vi "Test motor controll ability.vi"() -> ()   [LabVIEW 2016]
uses:
  Default PDO conf.ctl
  <vilib>/userdefined/High Color/nirio_resource_hc.ctl
  <vilib>/Platform/TimedLoop/XDataNode/timing_clust.ctl
  <vilib>/Platform/TimedLoop/XDataNode/nitl_modes.ctl
  <vilib>/Platform/TimedLoop/XDataNode/wakeup.ctl
  <vilib>/FPGAPlugInAG/cRIO-9033/niLvFpga_Open_cRIO-9033.vi
  <vilib>/rvi/interface/common/dynamic/niFpgaDynamicAddResources.vi
  <vilib>/CANopenLib/CANOPEN.llb/CANopen Emergency Create.vi
  <vilib>/CANopenLib/CANOPEN.llb/CANopen SDO Create.vi
  Set mode of operation.vi
  Set control mode.vi
  <vilib>/CANopenLib/CANOPEN.llb/CANopen SDO Close.vi
  Set Speed or Torque.vi
  Get Error.vi
  <vilib>/CANopenLib/CANOPEN.llb/CANopen Interface Close.vi
  <vilib>/rvi/interface/nirviOpenFPGA/nirviOpenFPGA.xnode
  FPGA Bitfiles/project_FPGATarget_FPGAMain_kDJZXzfRsH0.lvbitx
  Program Files (x86)/National Instruments/LabVIEW 2016/examples/robotics/EPOS2 CANOpen Driver/FPGA/FPGA Main.vi
  <vilib>/Platform/TimedLoop/XDataNode/XDataNode.xnode
  <vilib>/Platform/TimedLoop/XDataNode/XDNodeRunTimeDep.lvlib
panel:
  out "x+1":u16
  out "Used Node ID":u8 min=1 max=127 step=1
  in  "Node ID Left":u8=1 min=1 max=127 step=1
  in  "?":enum32{"Setup", "Operation", "Debug"}(tab)
  in  "Mode of operation":i8(ring)=9 items=["Induction VF – testing purposes only"=-5, "Aligning rotor position"=-4, "Current stepper – testing purposes only "=-3, "Voltage stepper – testing purposes only"=-2, "Voltage constant angle – testing purposes only"=-1, "No mode"=0, "Cyclic sync position"=8, "Cyclic sync velocity"=9, "Cyclic sync torque"=10]
  in  "Control Mode":u8(ring)=2 items=["Velocity"=2, "Torque"=1]
  out "Waveform Chart":cluster{"Controller temp":u8, "Motor temp":u8}(graph)
  in  "Set":bool
  in  "Stop":bool
  out "Decoded PDO":T1 {"Status word" format="%b"}
  in  "Speed-Torque":i32(knob) scale=-200.0..200.0
  in  "error in (no error)":errorcluster
  out "PDO 1":u8[](array[numeric])
  out "PDO 2":u8[](array[numeric])
  out "PDO 3":u8[](array[numeric])
  out "PDO 4":u8[](array[numeric])
  out "error out":errorcluster
  out "Error code":u16 format="%x"
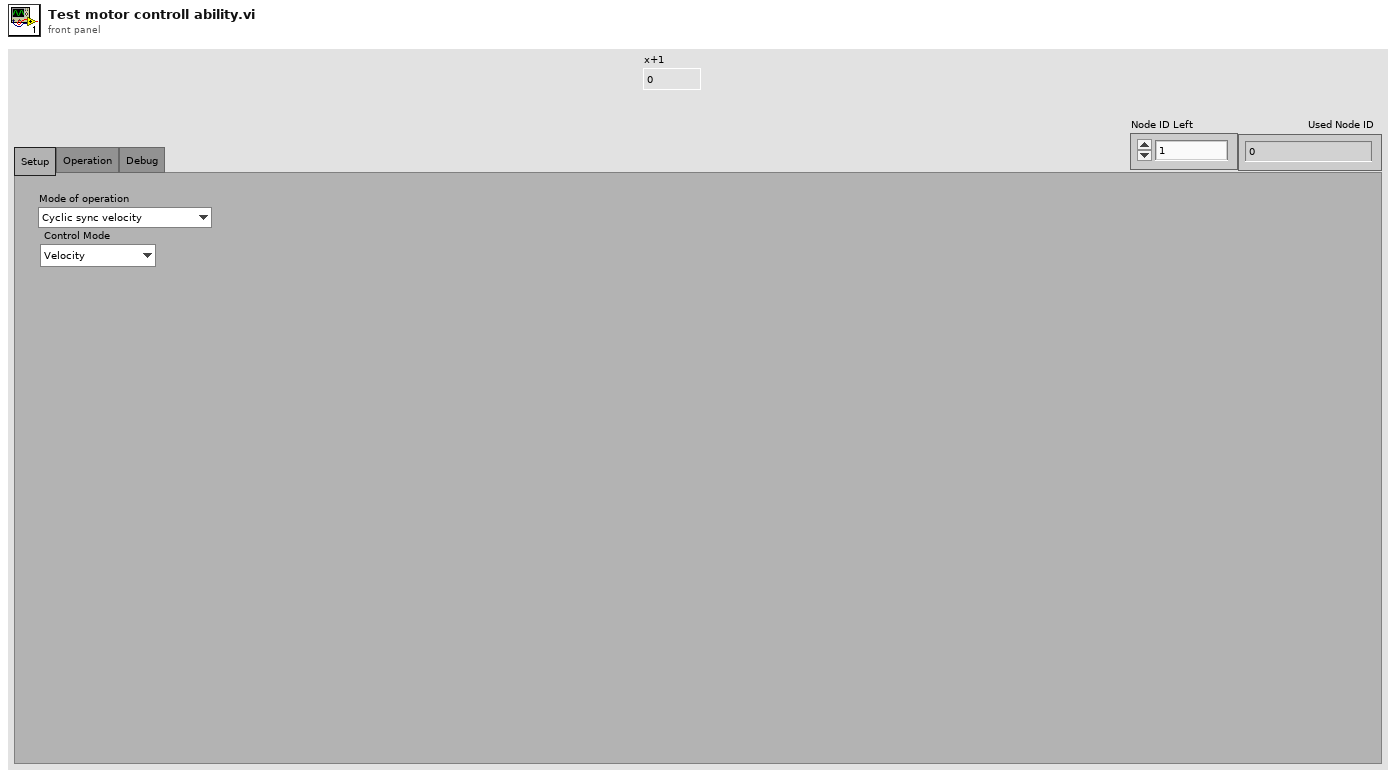
[diagram p1: front panel]
types:
  T1 = typedef "Default PDO conf.ctl" = cluster{"Status word":u16, "Position Actual Value":u32, "Torque Actual Value":u16, "Logic Power Supply Voltage":u16, "Current Demand":i32, "Controller temp":u8, "Motor temp":u8, "DC Link Voltage":u16, "Motor current actual value":u16, "Electrical angle":u16, "Phase A Current":u16, "Phase B Current":u16}
  T2 = typedef "nirio_resource_hc.ctl" = tag
  T3 = typedef "XDNodeRunTimeDep.lvlib/timing_clust.ctl" = cluster{"Expected End [f-1]":u64, "Actual End [f-1]":u64, "Finished Late? [f-1]":bool, "Expected End [i-1]":u64, "Actual End [i-1]":u64, "Finished Late? [i-1]":bool, "Expected Start [i]":u64, "Actual Start [i]":u64, "Expected Start [f]":u64, "Actual Start [f]":u64, "Source Name":string, "Structure Name":string, "Period":i64, "Deadline":i64, "Offset":i64, "Start":i64, "Priority":i32, "Timeout":i32, "Mode":T4, "Wakeup Reason":T5, "Error":errorcluster, "Source Type":string, "Secondary Source Type":string, "Global End Time":u64, "Global Start Time":u64, "Frame Duration":u64, "Iteration Duration":u64, "Assigned CPU":i32, "I/O Scan Engine Mode":u32}
  T4 = typedef "XDNodeRunTimeDep.lvlib/nitl_modes.ctl" = enum32{"No Change", "Process missed periods, maintain original phase", "Discard missed periods, maintain original phase", "Process missed periods, ignore original phase", "Discard missed periods, ignore original phase"}
  T5 = typedef "XDNodeRunTimeDep.lvlib/wakeup.ctl" = enum32{"Normal", "Aborted", "Asynchronous wakeup", "Timing source error", "Timed loop error", "Timeout"}
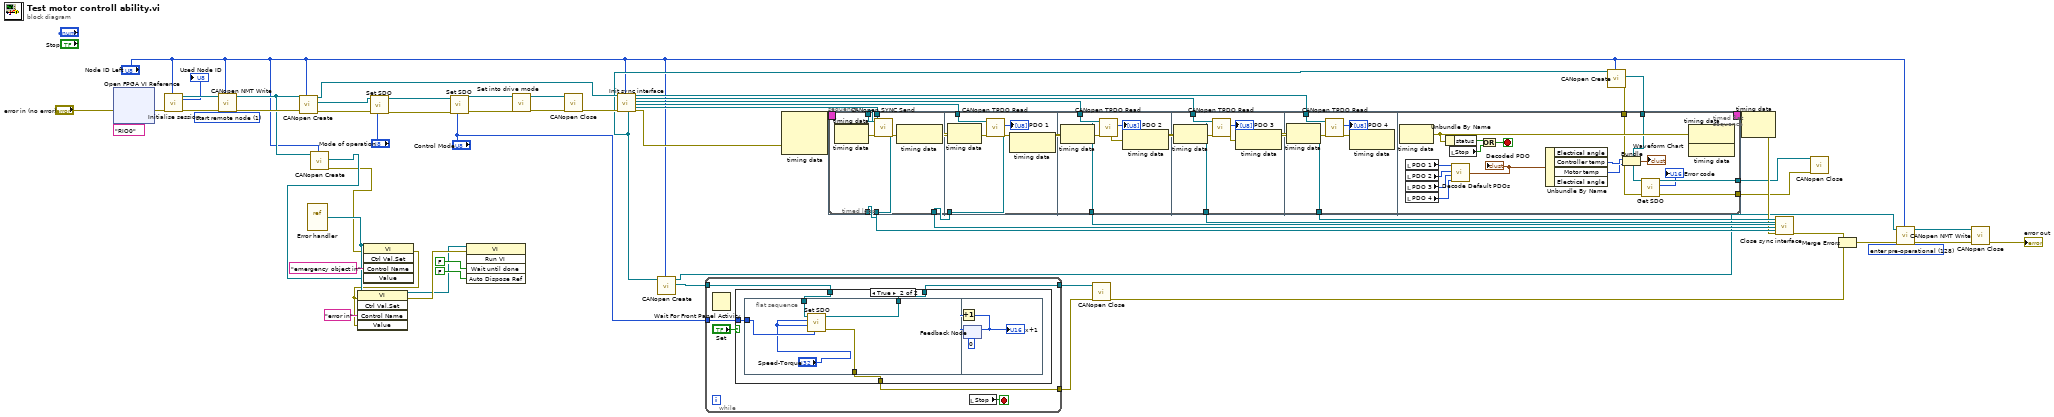
[diagram p0: block diagram]
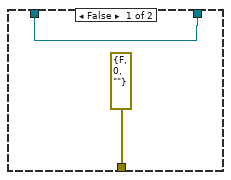
[diagram p2: hidden frame]
diagram:
  w51 = u16 1 items=["start remote node"=1, "stop remote node"=2, "enter pre-operational"=128, "reset node"=129, "reset communication"=130] ("command")
  w57 = u16 128 items=["start remote node"=1, "stop remote node"=2, "enter pre-operational"=128, "reset node"=129, "reset communication"=130] ("command")
  n1 = xnode ("Open FPGA VI Reference")("error in"="error in (no error)", "resource name"=T2 "RIO0") -> ("error out"=w61:errorcluster)  [unwired: 1 out]
  n2 = call "Initialise session.vi"("Node ID"="Node ID Left", "error in"=w61) -> ("error out"=w53:errorcluster, "interface object out"=w52:refnum<k20>, "Used Node ID"=→"Used Node ID":u8)  [unwired: 7 in]
  n3 = call <vilib>:"CANopen NMT Write.vi"("node-ID (0)"="Node ID Left", "error in (no error)"=w53, "command"=w51, "interface object in"=w52) -> ("error out"=w50:errorcluster, "interface object out"=w33:refnum<k20>)  [unwired: 6 in]
  n4 = call-poly <vilib>:"CANopen Create.vi"("node-ID"="Node ID Left", "error in (no error)"=w50, "interface object in"=w33) -> ("error out"=w29:errorcluster, "SDO object out"=w28:refnum<k20>, "interface object out"=w40:refnum<k20>)  [unwired: 6 in]
  n5 = vi-ref "Error handler.vi"() -> (w18:refnum<vi>)
  n6 = call-poly <vilib>:"CANopen Create.vi"("node-ID"="Node ID Left", "interface object in"=w33) -> ("error out"=w13:errorcluster, "emergency object out"=w14:refnum<k20>)  [unwired: 7 in, 1 out]
  n7 = invoke class="VI" method="Ctrl Val.Set"(reference=w18, error in=w13, "Control Name"="emergency object in", "Value"=w14) -> (error out=w17:errorcluster)  [unwired: 1 in, 4 out]
  n8 = invoke class="VI" method="Ctrl Val.Set"(reference=w18, error in=w17, "Control Name"="error in", "Value"=w17) -> (reference out=w15:refnum<vi>, error out=w16:errorcluster)  [unwired: 1 in, 3 out]
  n9 = call-poly "Set SDO.vi"("Mode of operation"="Mode of operation", "error in (no error)"=w29, "SDO object in"=w28) -> ("error out"=w26:errorcluster, "SDO object out"=w27:refnum<k20>)  [unwired: 6 in, 1 out]
  n10 = call-poly "Set SDO.vi"("Control Mode"="Control Mode", "error in (no error)"=w26, "SDO object in"=w27) -> ("error out"=w25:errorcluster, "SDO object out"=w24:refnum<k20>)  [unwired: 6 in, 1 out]
  n11 = invoke class="VI" method="Run VI"(reference=w15, error in=w16, "Wait until done"=FALSE ("Wait Until Done"), "Auto Dispose Ref"=FALSE ("Auto Dispose Reference")) -> ()  [unwired: 1 in, 5 out]
  n12 = call "Set into drive mode.vi"("error in (no error)"=w25, "SDO object in"=w24) -> ("error out"=w49:errorcluster, "SDO object out"=w48:refnum<k20>)  [unwired: 8 in]
  n13 = call-poly <vilib>:"CANopen Close.vi"("error in (no error)"=w49, "SDO object in"=w48) -> ("error out"=w41:errorcluster)  [unwired: 9 in]
  n14 = call "Init sync interface.vi"("interface object in"=w40, "error in (no error)"=w41, "node-ID"="Node ID Left") -> ("interface object out"=w8:refnum<k20>, "TPDO 4 object out"=w7:refnum<k20>, "TPDO 3 object out"=w43:refnum<k20>, "TPDO 2 object out"=w44:refnum<k20>, "TPDO 1 object out"=w45:refnum<k20>, "SYNC object out"=w46:refnum<k20>, "error out"=w42:errorcluster)  [unwired: 10 in]
  n15 = call-poly <vilib>:"CANopen Create.vi"("node-ID"="Node ID Left", "interface object in"=w8) -> ("SDO object out"=w3:refnum<k20>, "interface object out"=w30:refnum<k20>)  [unwired: 7 in, 1 out]
  n16 = while {
    tunnel: [w66] -> w5
    tunnel: w3 -> [w65]
    tunnel: [w64] -> w4
    tunnel: "Control Mode" -> [w63]
    stop <- w68 stop-if-true
    n17 = Wait For Front Panel Activity() -> ()  [unwired: 3 in, 1 out]
    n18 = case shown="True" "Set" {
      tunnel: [errorcluster {"status"=FALSE, "code"=0, "source"=""} ("error out") w74] -> w66
      tunnel: w65 -> [w69 w72]
      tunnel: [w69 w73] -> w64
      tunnel: w63 -> [_ w71]
      frame False {
      }
      frame True {
        n19 = flat-sequence {
          tunnel: [w78] -> w73
          tunnel: [w77] -> w74
          tunnel: w72 -> [w79]
          tunnel: w71 -> [w76]
          frame #0 {
            n20 = call-poly "Set SDO.vi"("Control Mode"=w76, "Speed"="Speed-Torque", "Torque"="Speed-Torque", "SDO object in"=w79) -> ("error out"=w77:errorcluster, "SDO object out"=w78:refnum<k20>)  [unwired: 5 in, 1 out]
          }
          frame #1 {
            n21 = feedback #1(u16 0) -> (w81:u16)
            n22 = Increment(x=w81) -> (x+1=w80:u16)
            "x+1" <- w80
            n23 = feedback-in #1(w80) -> ()
          }
        }
      }
    }
    n24 = local read "Stop"() -> (w68:bool)
  }
  n25 = node-c288(w42) -> (w60:T3)  [unwired: 2 in]
  n26 = call-poly <vilib>:"CANopen Close.vi"("error in (no error)"=w5, "SDO object in"=w4) -> ("error out"=w47:errorcluster)  [unwired: 9 in]
  n27 = call-poly <vilib>:"CANopen Create.vi"("node-ID"="Node ID Left", "interface object in"=w8) -> ("error out"=w12:errorcluster, "SDO object out"=w11:refnum<k20>)  [unwired: 7 in, 1 out]
  n28 = timed-loop {
    timing: w60 -> [_]
    timing-out: [_] -> w59
    tunnel: w46 -> [w96]
    tunnel: w45 -> [w95]
    tunnel: [w94] -> w36
    tunnel: w44 -> [w93]
    tunnel: [w92] -> w37
    tunnel: w43 -> [w91]
    tunnel: w7 -> [w90]
    tunnel: [w89] -> w39
    tunnel: [w88] -> w38
    tunnel: [w87] -> w35
    tunnel: w11 -> [w86]
    tunnel: w12 -> [w85]
    tunnel: [w84] -> w10
    tunnel: [w83] -> w9
    stop <- w169 stop-if-true
    n29 = timed-sequence {
      timing: _ -> [_]
      timing-out: _ -> [_]
      tunnel: w96 -> [w110]
      tunnel: w95 -> [w109]
      tunnel: [w108] -> w94
      tunnel: w93 -> [w107]
      tunnel: [w106] -> w92
      tunnel: w91 -> [w105]
      tunnel: w90 -> [w104]
      tunnel: [w103] -> w89
      tunnel: [w102] -> w88
      tunnel: [w101] -> w87
      tunnel: w86 -> [w100]
      tunnel: w85 -> [w99]
      tunnel: [w98] -> w84
      tunnel: [w97] -> w83
      n30 = timed-flat-sequence {
        tunnel: w110 -> [w114]
        tunnel: [w111] -> w101
        tunnel: w109 -> [w124]
        tunnel: [w123] -> w108
        tunnel: w107 -> [w131]
        tunnel: [w130] -> w106
        tunnel: w105 -> [w141]
        tunnel: [w140] -> w102
        tunnel: w104 -> [w152]
        tunnel: [w151] -> w103
        tunnel: w100 -> [w167]
        tunnel: w99 -> [w164]
        tunnel: [w166] -> w98
        tunnel: [w165] -> w97
        frame #0 {
          n31 = node-c288() -> (w113:errorcluster)  [unwired: 1 in]
          n32 = call <vilib>:"CANopen SYNC Send.vi"("error in (no error)"=w113, "SYNC object in"=w114) -> ("error out"=w112:errorcluster, "SYNC object out"=w111:refnum<k20>)  [unwired: 8 in]
          n33 = node-c288(w112) -> ()  [unwired: 1 out]
        }
        frame #1 {
          n34 = node-c288() -> (w122:errorcluster)  [unwired: 1 in]
          n35 = call <vilib>:"CANopen TPDO Read.vi"("error in (no error)"=w122, "TPDO object in"=w124) -> ("error out"=w121:errorcluster, "data"=→"PDO 1":u8[], "TPDO object out"=w123:refnum<k20>)  [unwired: 5 in, 2 out]
          n36 = node-c288(w121) -> ()  [unwired: 1 out]
        }
        frame #2 {
          n37 = node-c288() -> (w133:errorcluster)  [unwired: 1 in]
          n38 = call <vilib>:"CANopen TPDO Read.vi"("error in (no error)"=w133, "TPDO object in"=w131) -> ("error out"=w132:errorcluster, "data"=→"PDO 2":u8[], "TPDO object out"=w130:refnum<k20>)  [unwired: 5 in, 2 out]
          n39 = node-c288(w132) -> ()  [unwired: 1 out]
        }
        frame #3 {
          n40 = node-c288() -> (w143:errorcluster)  [unwired: 1 in]
          n41 = call <vilib>:"CANopen TPDO Read.vi"("error in (no error)"=w143, "TPDO object in"=w141) -> ("error out"=w142:errorcluster, "data"=→"PDO 3":u8[], "TPDO object out"=w140:refnum<k20>)  [unwired: 5 in, 2 out]
          n42 = node-c288(w142) -> ()  [unwired: 1 out]
        }
        frame #4 {
          n43 = node-c288() -> (w153:errorcluster)  [unwired: 1 in]
          n44 = call <vilib>:"CANopen TPDO Read.vi"("error in (no error)"=w153, "TPDO object in"=w152) -> ("error out"=w150:errorcluster, "data"=→"PDO 4":u8[], "TPDO object out"=w151:refnum<k20>)  [unwired: 5 in, 2 out]
          n45 = node-c288(w150) -> ()  [unwired: 1 out]
        }
        frame #5 {
          n46 = node-c288() -> (w172:errorcluster)  [unwired: 1 in]
          n47 = local read "PDO 1"() -> (w176:u8[])
          n48 = local read "PDO 2"() -> (w175:u8[])
          n49 = local read "PDO 3"() -> (w174:u8[])
          n50 = local read "PDO 4"() -> (w173:u8[])
          n51 = Unbundle By Name(w172) -> ("status"=w171:bool)
          n52 = local read "Stop"() -> (w170:bool)
          n53 = call "Decode Default PDOs.vi"("PDO 4"=w173, "PDO 3"=w174, "PDO 2"=w175, "PDO 1"=w176) -> ("Decoded PDO"=w168:T1)
          "Decoded PDO" <- w168
          n54 = Or(x=w171, y=w170) -> (x .or. y?=w169:bool)
          n55 = Unbundle By Name(w168) -> ("Controller temp"=w161:u8, "Motor temp"=w160:u8)  [unwired: 2 out]
          n56 = Bundle("Controller temp"=w161, "Motor temp"=w160) -> (→"Waveform Chart":cluster{"Controller temp":u8, "Motor temp":u8})  [unwired: 1 in]
          n57 = call-poly "Get SDO.vi"("error in (no error)"=w164, "SDO object in"=w167) -> ("error out"=w165:errorcluster, "Error code"=→"Error code":u16, "SDO object out"=w166:refnum<k20>)  [unwired: 5 in, 2 out]
          n58 = node-c288(w172) -> ()  [unwired: 1 out]
        }
      }
    }
    n59 = node-c288() -> ()  [unwired: 1 in, 1 out]
    n60 = node-c288() -> ()  [unwired: 1 in, 1 out]
  }
  n61 = node-c288(w59) -> (w31:errorcluster)
  n62 = call "Close sync interface.vi"("TPDO 4 object in"=w39, "TPDO 3 object in"=w38, "TPDO 2 object in"=w37, "TPDO 1 object in"=w36, "SYNC object in"=w35, "error in (no error)"=w31) -> ("error out"=w34:errorcluster)  [unwired: 13 in]
  n63 = call-poly <vilib>:"CANopen Close.vi"("error in (no error)"=w9, "SDO object in"=w10) -> ()  [unwired: 9 in, 1 out]
  n64 = Merge Errors(w34, w47) -> (w32:errorcluster)
  n65 = call <vilib>:"CANopen NMT Write.vi"("node-ID (0)"="Node ID Left", "error in (no error)"=w32, "command"=w57, "interface object in"=w30) -> ("error out"=w55:errorcluster, "interface object out"=w56:refnum<k20>)  [unwired: 6 in]
  n66 = call-poly <vilib>:"CANopen Close.vi"("error in (no error)"=w55, "interface object in"=w56) -> ("error out"=→"error out":errorcluster)  [unwired: 9 in]
